vi "ATMonochromator_logEvent_settingVersions.vi"(8 "error in (no error)":errorcluster, 11 "logevent_settingVersions_Ctl":T1) -> (0 "error out":errorcluster, 2 "function return":i32, 3 "logevent_settingVersions_Ctl out":T1)   [LabVIEW 2016, in "SALLV_ATMonochromator.lvlib"]
doc: "int ATMonochromator_shm_logEvent_settingVersionsLV(ATMonochromator_logevent_settingVersionsLV *logevent_settingVersions_Ctl );"
uses:
  SALLV_ATMonochromator.lvlib
  DataTypes/logevent_settingVersions.ctl
  SALLV_ATMonochromator.so
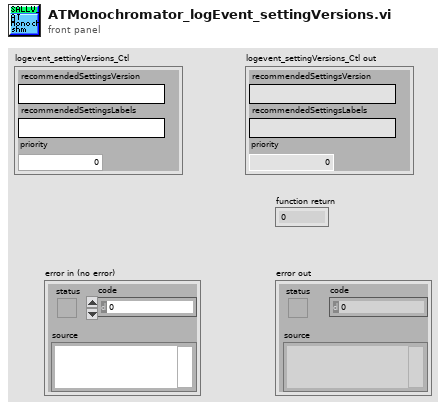
[diagram p1: front panel]
types:
  T1 = typedef "SALLV_ATMonochromator.lvlib/logevent_settingVersions.ctl" = cluster{"recommendedSettingsVersion":string, "recommendedSettingsLabels":string, "priority":i32}
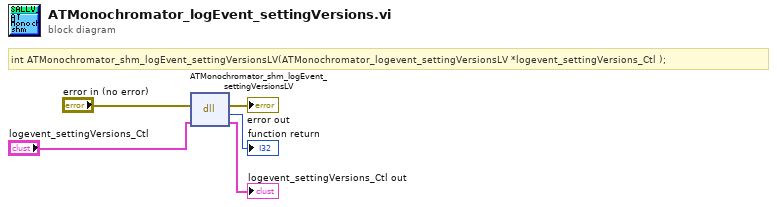
[diagram p0: block diagram]
diagram:
  # "int ATMonochromator_shm_logEvent_settingVersionsLV(ATMonochromator_logevent_settingVersionsLV *logevent_settingVersions_Ctl );"
  n1 = dll-call lib="home/harini/tcs/SALLV_ATMonochromator/SALLV_ATMonochromator.*" fn="ATMonochromator_shm_logEvent_settingVersionsLV"(error in="error in (no error)", "logevent_settingVersions_Ctl"="logevent_settingVersions_Ctl") -> (error out=→"error out":errorcluster, →"function return":i32, "logevent_settingVersions_Ctl"=→"logevent_settingVersions_Ctl out":T1)  [unwired: 2 in, 1 out]
